vi "Area.vi"(8 "error in (no error)":errorcluster, 11 "Rectangle in":refnum<class "Rectangle.lvclass">) -> (0 "error out":errorcluster, 2 "rect":T1, 3 "Rectangle out":refnum<class "Rectangle.lvclass">)   [LabVIEW 2021, in "Picture2D.lvlib" / "Rectangle.lvclass"]
uses:
  Rectangle.lvclass
  Point/Point.lvclass
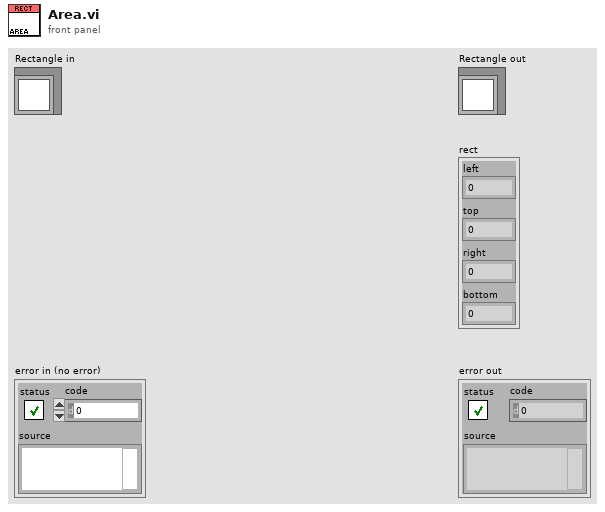
[diagram p1: front panel]
types:
  T1 = cluster{"left":i16, "top":i16, "right":i16, "bottom":i16}
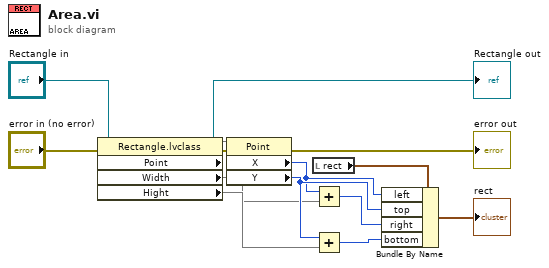
[diagram p0: block diagram]
diagram:
  n1 = property class="Rectangle.lvclass"(reference="Rectangle in", error in="error in (no error)") -> (reference out=→"Rectangle out":refnum<class "Rectangle.lvclass">, error out=w2:errorcluster, "Point"=w9, "Width"=w3, "Hight"=w7)
  n2 = property class="Point"(reference=w9, error in=w2) -> (error out=→"error out":errorcluster, "X"=w5:i16, "Y"=w6:i16)  [unwired: 1 out]
  n3 = local read "rect"() -> (w11:T1)
  n4 = Add(x=w5, y=w3) -> (x+y=w4:i16)
  n5 = Add(x=w6, y=w7) -> (x+y=w8:i16)
  n6 = Bundle By Name(cluster=w11, "left"=w5, "top"=w6, "right"=w4, "bottom"=w8) -> (→"rect":T1)
